vi "Open Event Arguments.vi"(8 "error in (no error)":errorcluster, 11 "VI Refnum":refnum<vi>) -> (0 "error out":errorcluster)   [LabVIEW 2019, in "Panther Dashboard.lvlib"]
uses:
  Panther Dashboard.lvlib
  <vilib>/Utility/traverseref.llb/TRef TravTarget.ctl
  <vilib>/Utility/traverseref.llb/VI Scripting - Traverse.lvlib
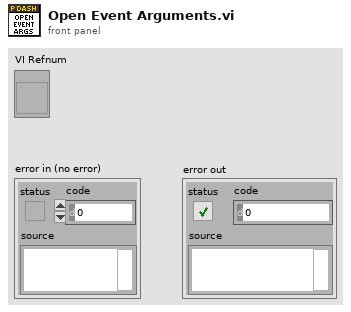
[diagram p1: front panel]
types:
  T1 = typedef "TRef TravTarget.ctl" = enum16{"FP", "BD", "Other"}
  T2 = enum32{"not a typedef", "typedef", "strict typedef", "class private data"}
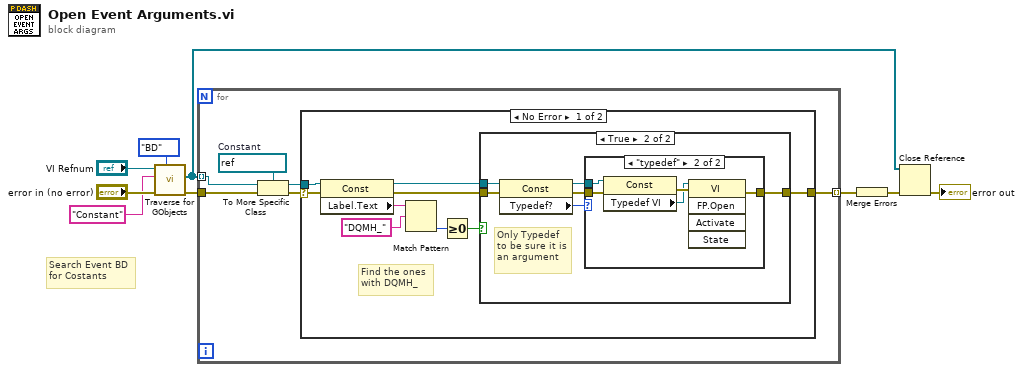
[diagram p0: block diagram]
diagram:
  # "Search Event BD\nfor Costants"
  n1 = call <vilib>:"Traverse for GObjects.vi"("Traverse Target"=TRef_TravTarget."BD", "error in (no error)"="error in (no error)", "Class Name"="Constant", "VI Refnum"="VI Refnum") -> ("error out"=w7:errorcluster, "References"=w3:refnum<vi>[])  [unwired: 4 in, 2 out]
  n2 = for {
    tunnel: w3 -> [w10] mode=indexing
    tunnel: [w14] -> w2 mode=indexing
    tunnel: w7 -> [w13]
    w11 = refnum<vi> refnum  # Constant
    n3 = To More Specific Class(target class=w11, reference=w10, error in=w13) -> (specific class reference=w12:refnum<vi>, error out=w15:errorcluster)
    n4 = case shown="No Error" w15 {
      selector: w15 -> [w24 w38]
      tunnel: w12 -> [w21 _]
      tunnel: [w22 w38] -> w14
      frame No Error {
        # "Find the ones\nwith DQMH_"
        n5 = property class="Const"(reference=w21, error in=w24) -> (reference out=w16:refnum<vi>, error out=w23:errorcluster, "Label.Text"=w20:string)
        n6 = Match Pattern(string=w20, regular expression="DQMH_") -> (offset past match=w18:i32)  [unwired: 1 in, 3 out]
        n7 = Greater Or Equal To 0?(x=w18) -> (x >= 0?=w17:bool)
        n8 = case shown="True" w17 {
          tunnel: w16 -> [_ w28]
          tunnel: w23 -> [w25 w31]
          tunnel: [w25 w29] -> w22
          frame False {
          }
          frame True {
            # "Only Typedef\nto be sure it is\nan argument"
            n9 = property class="Const"(reference=w28, error in=w31) -> (reference out=w26:refnum<vi>, error out=w30:errorcluster, "Typedef?"=w27:T2)
            n10 = case shown="\"typedef\"" w27 {
              tunnel: w26 -> [_ w35]
              tunnel: [w32 w37] -> w29
              tunnel: w30 -> [w32 w33]
              frame "not a typedef", Default {
              }
              frame "typedef" {
                n11 = property class="Const"(reference=w35, error in=w33) -> (error out=w36:errorcluster, "Typedef VI"=w34:refnum<vi>)  [unwired: 1 out]
                n12 = invoke class="VI" method="FP.Open"(reference=w34, error in=w36) -> (error out=w37:errorcluster)  [unwired: 3 in, 4 out]
              }
            }
          }
        }
      }
      frame Error {
      }
    }
  }
  n13 = Merge Errors(w2) -> (w9:errorcluster)
  n14 = Close Reference(reference=w3, error in (no error)=w9) -> (error out=→"error out":errorcluster)
